vi "Main.vi"() -> ()   [LabVIEW 2015]
doc: "This template is for the Queued Message Handler design pattern.\n\nThe Event Handling Loop generates messages based on user interface actions.\n\nThe Message Handling Loop processes messages generated by the Event Handling Loop, or by other messages. The messages are string values, so new messages can be added easily to the Message Cases case structure in the Message Handling Loop. Each message cluster can also provide an optional value for Message Data, which is a variant that can be converted to whatever message-specific data is required."
uses:
  controls/UI Data.ctl
  support/Message Queue/Message Queue.lvlib
  support/User Event - Stop/User Event - Stop.lvlib
  support/Boiler System Globals.vi
  Boiler/Boiler.lvlib
  support/Notifiers/Notifiers.ctl
panel:
  out "Display <Replace Me>":string
  in  "Do Something Else <Replace Me>":bool
  in  "Do Something <Replace Me>":bool
  in  "Stop Button":bool
  # "These controls have associated \"Value Changed\" events configured in the Event Structure on the diagram.\n\nReplace them (and reconfigure the Event Structure) with the controls you need for your application."
  # "This template is for the Queued Message Handler design pattern.\n\nSee the block diagram for more information on how to use this template."
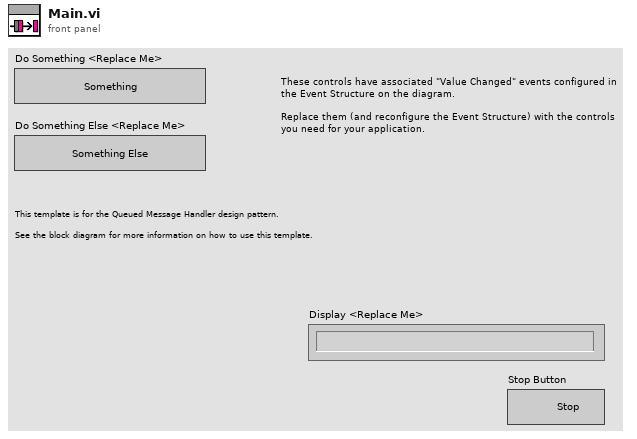
[diagram p1: front panel]
types:
  T1 = typedef "Notifiers.ctl" = cluster{"Handshake":refnum<notifier>, "Flame level":refnum<notifier>, "Controller exit":refnum<notifier>, "Boiler exit":refnum<notifier>}
  T2 = typedef "UI Data.ctl" = cluster{"Boolean <Replace Me>":bool, "String <Replace Me>":string, "Numeric <Replace Me>":dbl, "Do Something Ref":refnum<vi>, "Do Something Else Ref":refnum<vi>, "Data Display Ref":refnum<vi>, "Stop Button Ref":refnum<vi>}
  T3 = typedef "Message Queue.lvlib/All Message Queues.ctl" = cluster{"MHL":refnum<queue>, "Boiler Controller":refnum<queue>, "Boiler":refnum<queue>}
  T4 = enum32{"invalid app kind", "Development System", "Run Time System", "Student Edition", "Embedded LabVIEW", "Evaluation", "Custom"}
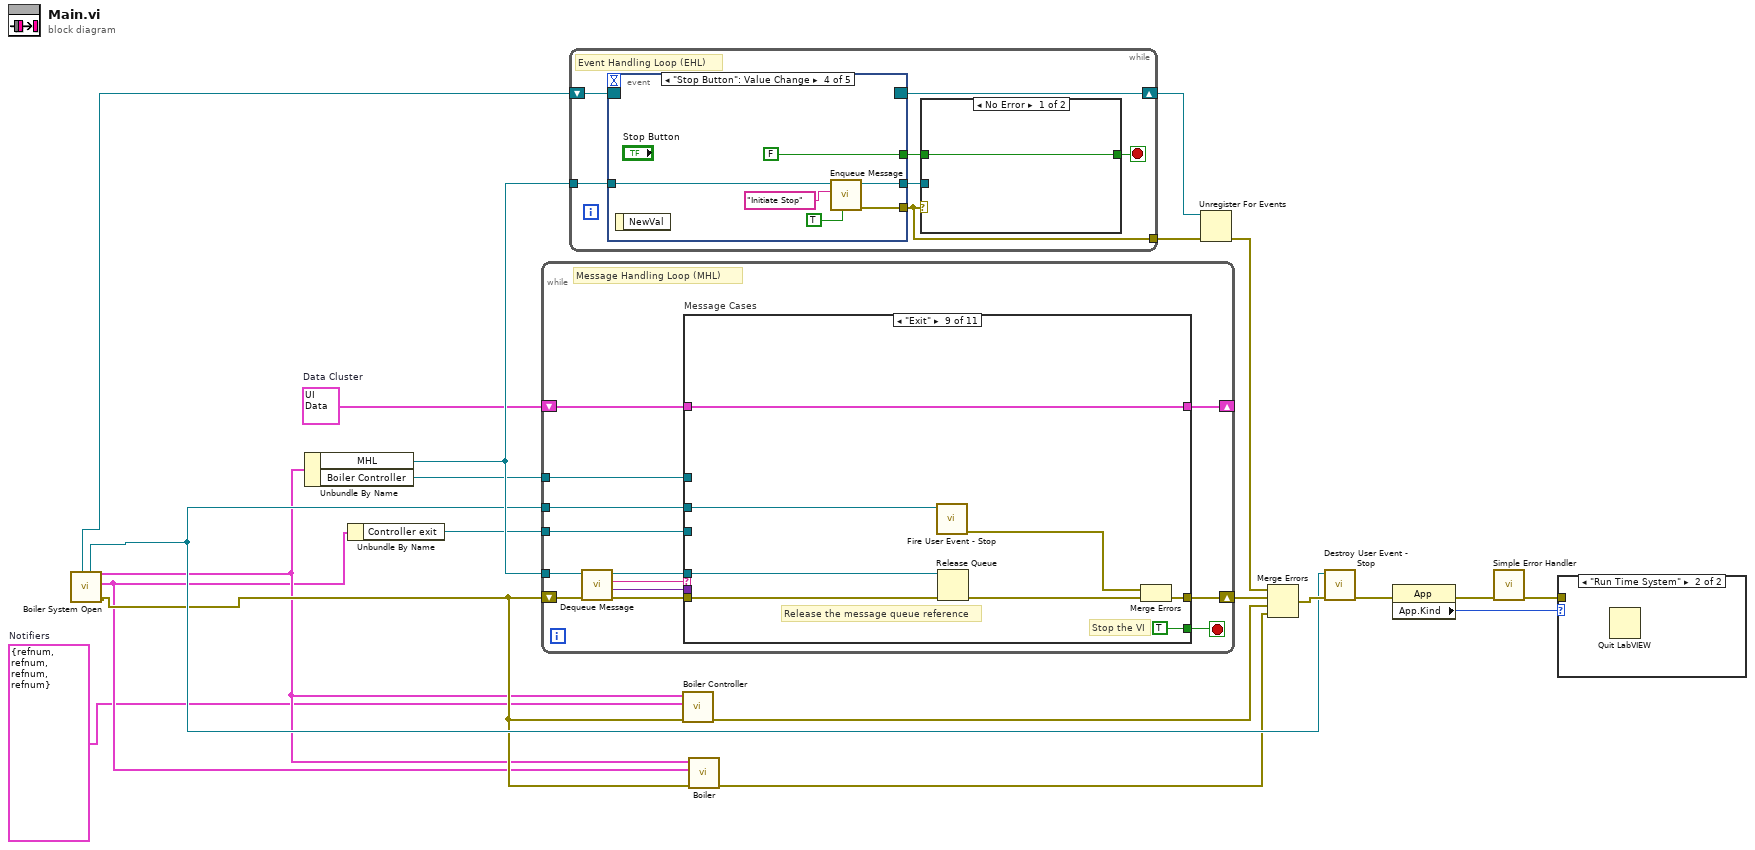
[diagram p0: block diagram]
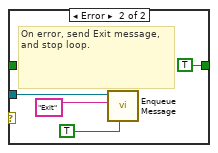
[diagram p3: hidden frame]
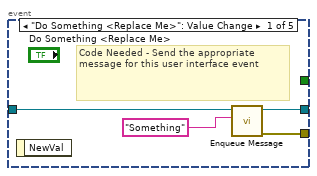
[diagram p4: hidden frame]
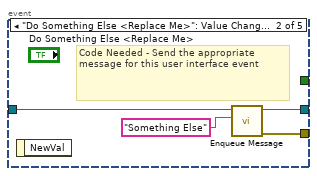
[diagram p5: hidden frame]
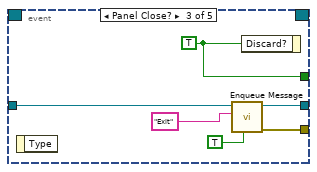
[diagram p6: hidden frame]
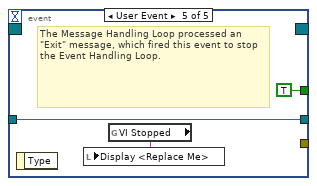
[diagram p7: hidden frame]
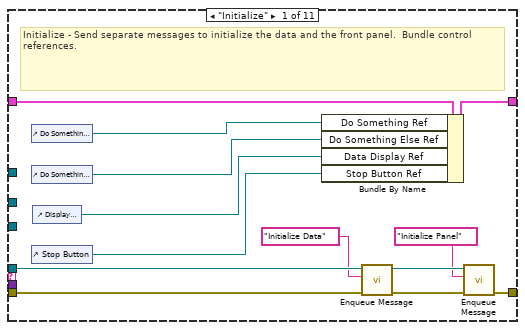
[diagram p8: hidden frame]
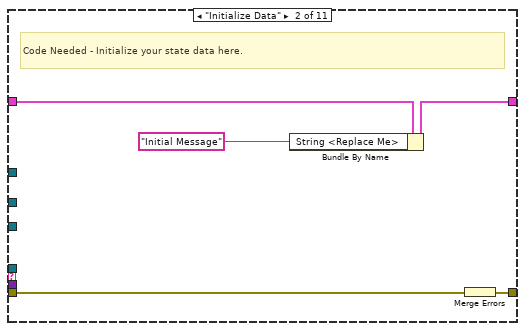
[diagram p9: hidden frame]
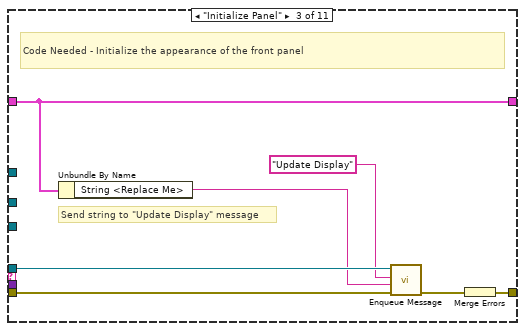
[diagram p10: hidden frame]
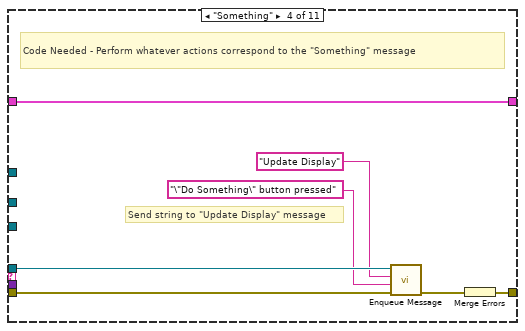
[diagram p11: hidden frame]
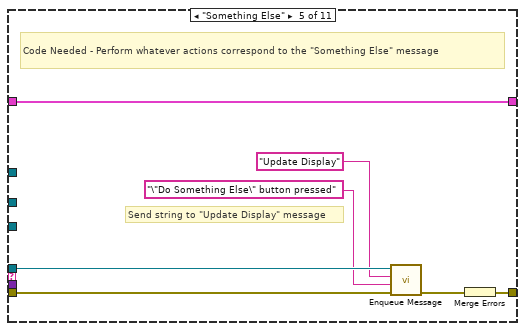
[diagram p12: hidden frame]
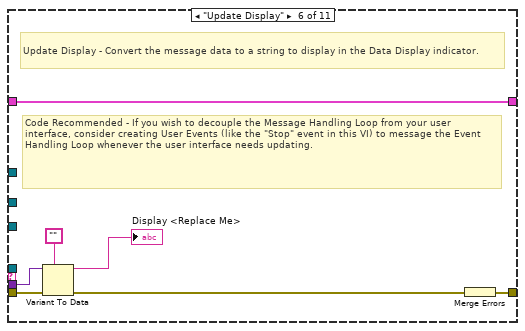
[diagram p13: hidden frame]
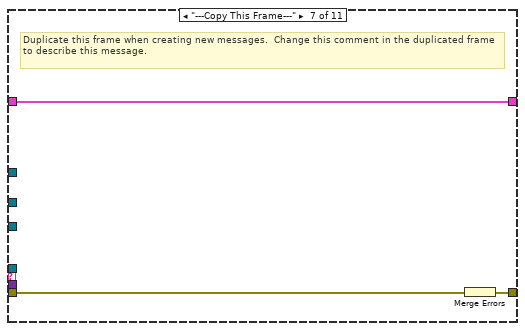
[diagram p14: hidden frame]
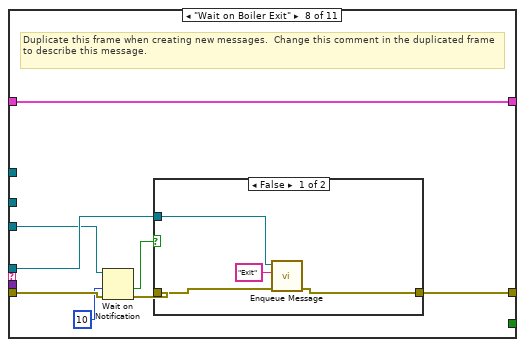
[diagram p15: hidden frame]
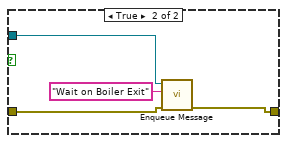
[diagram p16: hidden frame]
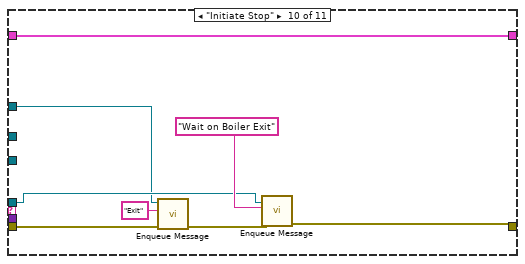
[diagram p17: hidden frame]
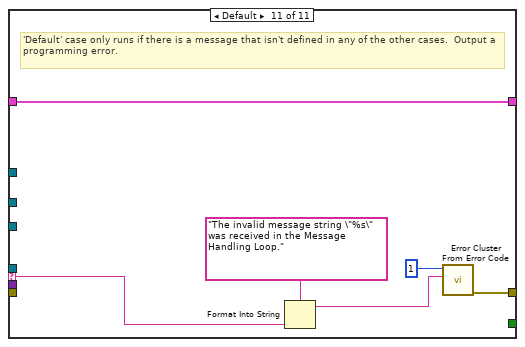
[diagram p18: hidden frame]
diagram:
  w1 = T1 {"Handshake"=refnum, "Flame level"=refnum, "Controller exit"=refnum, "Boiler exit"=refnum}  # Notifiers
  w14 = T2 {"Boolean <Replace Me>"=TRUE, "String <Replace Me>"="", "Numeric <Replace Me>"=0.0, "Do Something Ref"=refnum, "Do Something Else Ref"=refnum, "Data Display Ref"=refnum, "Stop Button Ref"=refnum}  # Data Cluster
  n1 = call "Boiler System Open.vi"() -> ("error out 2"=w6:errorcluster, "Notifiers"=w3:T1, "Message Queues out 2"=w5:T3, "User Event - Stop 2"=w7:refnum<user-event>, "Stop Event Registration Refnum 2"=w8:refnum<event-registration>)  [unwired: 7 in]
  n2 = Unbundle By Name(w5) -> ("MHL"=w20:refnum<queue>, "Boiler Controller"=w12:refnum<queue>)
  n3 = Unbundle By Name(w3) -> ("Controller exit"=w2:refnum<notifier>)
  n4 = while {
    tunnel: w20 -> [w24]
    shift-right: [w33] -> _
    shift-left: w14 -> [w34]
    tunnel: w7 -> [w30]
    shift-right: [w31] -> w21
    shift-left: w6 -> [w29]
    tunnel: w12 -> [w23]
    tunnel: w2 -> [w22]
    stop <- w32 stop-if-true
    # "Message Handling Loop (MHL)"
    n5 = call "Dequeue Message.vi"("error in (no error)"=w29, "Message Queue"=w24) -> ("error out"=w28:errorcluster, "Message Data"=w26:variant, "Message"=w27:string, "dup Message Queue"=w25:refnum<queue>)  [unwired: 6 in]
    n6 = case "Message Cases" shown="\"Exit\"" w27 {
      selector: w27 -> [_ _ _ _ _ _ _ _ _ _ w119]
      tunnel: w25 -> [w43 _ w56 w62 w69 _ _ w89 w107 w109 _]
      tunnel: w28 -> [w46 w52 w57 w64 w71 w78 w83 w88 w100 w114 _]
      tunnel: [w47 w48 w58 w65 w72 w79 w81 w90 w103 w112 w117] -> w31
      tunnel: w34 -> [w40 w51 w59 w66 w73 w80 w82 w91 w106 w115 w121]
      tunnel: [w39 w50 w59 w66 w73 w80 w82 w91 w106 w115 w121] -> w33
      tunnel: [_ _ _ _ _ _ _ _ TRUE _ _] -> w32
      tunnel: w26 -> [_ _ _ _ _ w77 _ _ _ _ _]
      tunnel: w30 -> [_ _ _ _ _ _ _ _ w102 _ _]
      tunnel: w23 -> [_ _ _ _ _ _ _ _ _ w108 _]
      tunnel: w22 -> [_ _ _ _ _ _ _ w85 _ _ _]
      frame "Initialize" {
        # "Initialize - Send separate messages to initialize the data and the front panel.  Bundle control references."
        n7 = control-ref of="Do Something <Replace Me>"() -> (w38:refnum<vi>)
        n8 = control-ref of="Do Something Else <Replace Me>"() -> (w37:refnum<vi>)
        n9 = control-ref of="Stop Button"() -> (w35:refnum<vi>)
        n10 = control-ref of="Display <Replace Me>"() -> (w36:refnum<vi>)
        n11 = Bundle By Name(cluster=w40, "Do Something Ref"=w38, "Do Something Else Ref"=w37, "Data Display Ref"=w36, "Stop Button Ref"=w35) -> (w39:T2)
        n12 = call "Enqueue Message.vi"("error in (no error)"=w46, "Message"="Initialize Data", "Message Queue"=w43) -> ("error out"=w45:errorcluster, "dup Message Queue"=w44:refnum<queue>)  [unwired: 7 in]
        n13 = call "Enqueue Message.vi"("error in (no error)"=w45, "Message"="Initialize Panel", "Message Queue"=w44) -> ("error out"=w47:errorcluster)  [unwired: 7 in, 1 out]
      }
      frame "Initialize Data" {
        # "Code Needed - Initialize your state data here."
        n14 = Bundle By Name(cluster=w51, "String <Replace Me>"="Initial Message" ("Initial Message")) -> (w50:T2)
        n15 = Merge Errors(w52) -> (w48:errorcluster)
      }
      frame "Initialize Panel" {
        # "Send string to \"Update Display\" message"
        # "Code Needed - Initialize the appearance of the front panel"
        n16 = Unbundle By Name(w59) -> ("String <Replace Me>"=w53:string)
        n17 = call "Enqueue Message.vi"("error in (no error)"=w57, "Message Data"=w53, "Message"="Update Display", "Message Queue"=w56) -> ("error out"=w55:errorcluster)  [unwired: 6 in, 1 out]
        n18 = Merge Errors(w55) -> (w58:errorcluster)
      }
      frame "Something" {
        # "Send string to \"Update Display\" message"
        # "Code Needed - Perform whatever actions correspond to the \"Something\" message"
        n19 = call "Enqueue Message.vi"("error in (no error)"=w64, "Message Data"="\"Do Something\" button pressed" ("\"Do Something\" button pressed"), "Message"="Update Display", "Message Queue"=w62) -> ("error out"=w63:errorcluster)  [unwired: 6 in, 1 out]
        n20 = Merge Errors(w63) -> (w65:errorcluster)
      }
      frame "Something Else" {
        # "Send string to \"Update Display\" message"
        # "Code Needed - Perform whatever actions correspond to the \"Something Else\" message"
        n21 = call "Enqueue Message.vi"("error in (no error)"=w71, "Message Data"="\"Do Something Else\" button pressed" ("\"Do Something Else\" button pressed"), "Message"="Update Display", "Message Queue"=w69) -> ("error out"=w70:errorcluster)  [unwired: 6 in, 1 out]
        n22 = Merge Errors(w70) -> (w72:errorcluster)
      }
      frame "Update Display" {
        # "Code Recommended - If you wish to decouple the Message Handling Loop from your user interface, consider creating User Events (like the \"Stop\" event in this VI) to message the Event Handling Loop whenever the user interface needs updating."
        # "Update Display - Convert the message data to a string to display in the Data Display indicator."
        n23 = Variant To Data(error in=w78, type="", Variant=w77) -> (data=→"Display <Replace Me>":string, error out=w75:errorcluster)
        n24 = Merge Errors(w75) -> (w79:errorcluster)
      }
      frame "---Copy This Frame---" {
        # "Duplicate this frame when creating new messages.  Change this comment in the duplicated frame to describe this message."
        n25 = Merge Errors(w83) -> (w81:errorcluster)
      }
      frame "Wait on Boiler Exit" {
        # "Duplicate this frame when creating new messages.  Change this comment in the duplicated frame to describe this message."
        n26 = Wait on Notification(notifier=w85, timeout in ms (-1)=10, error in (no error)=w88) -> (timed out?=w84:bool, error out=w87:errorcluster)  [unwired: 1 in, 2 out]
        n27 = case shown="False" w84 {
          tunnel: w87 -> [w95 w99]
          tunnel: [w94 w98] -> w90
          tunnel: w89 -> [w92 w96]
          frame False {
            n28 = call "Enqueue Message.vi"("error in (no error)"=w95, "Message"="Exit", "Message Queue"=w92) -> ("error out"=w94:errorcluster)  [unwired: 7 in, 1 out]
          }
          frame True {
            n29 = call "Enqueue Message.vi"("error in (no error)"=w99, "Message"="Wait on Boiler Exit", "Message Queue"=w96) -> ("error out"=w98:errorcluster)  [unwired: 7 in, 1 out]
          }
        }
      }
      frame "Exit" {
        # "Stop the VI"
        # "Release the message queue reference"
        n30 = call "Fire User Event - Stop.vi"("User Event - Stop"=w102) -> ("error out"=w101:errorcluster)  [unwired: 10 in]
        n31 = Release Queue(queue=w107, error in (no error)=w100) -> (error out=w104:errorcluster)  [unwired: 1 in, 2 out]
        n32 = Merge Errors(w101, w104) -> (w103:errorcluster)
      }
      frame "Initiate Stop" {
        n33 = call "Enqueue Message.vi"("error in (no error)"=w114, "Message"="Exit", "Message Queue"=w108) -> ("error out"=w113:errorcluster)  [unwired: 7 in, 1 out]
        n34 = call "Enqueue Message.vi"("error in (no error)"=w113, "Message"="Wait on Boiler Exit", "Message Queue"=w109) -> ("error out"=w112:errorcluster)  [unwired: 7 in, 1 out]
      }
      frame Default {
        # "'Default' case only runs if there is a message that isn't defined in any of the other cases.  Output a programming error."
        n35 = Format Into String(format string="The invalid message string \"%s\" was received in the Message Handling Loop." ("Unknown Message Error Text"), w119) -> (resulting string=w116:string)  [unwired: 2 in, 1 out]
        n36 = call <vilib>:"Error Cluster From Error Code.vi"("error message (\"\")"=w116, "error code (0)"=1) -> ("error out"=w117:errorcluster)  [unwired: 7 in]
      }
    }
  }
  n37 = while {
    tunnel: w20 -> [w128]
    tunnel: [w124] -> w16
    shift-right: [w122] -> w15
    shift-left: w8 -> [w123]
    stop <- w126 stop-if-true
    # "Event Handling Loop (EHL)"
    n38 = event shown="[3] \"Stop Button\": Value Change" {
      selector: w123 -> [_ _ _ _ _]
      dyn-events: [_ _ _ _ _] -> w122
      timeout: _ -> [_ _ _ _ _]
      tunnel: [_ _ w147 FALSE ("Discard?") TRUE ("Discard?")] -> w127
      tunnel: w128 -> [w137 w141 w146 w153 w156]
      tunnel: [w136 w139 w145 w152 _] -> w124
      tunnel: [w135 w140 w144 w150 w156] -> w125
      event "Do Something <Replace Me>": Value Change {
        # "Code Needed - Send the appropriate message for this user interface event"
        n39 = event-data() -> ()  [unwired: 1 in, 1 out]
        n40 = call "Enqueue Message.vi"("Message"="Something", "Message Queue"=w137) -> ("error out"=w136:errorcluster, "dup Message Queue"=w135:refnum<queue>)  [unwired: 8 in]
      }
      event "Do Something Else <Replace Me>": Value Change {
        # "Code Needed - Send the appropriate message for this user interface event"
        n41 = event-data() -> ()  [unwired: 1 in, 1 out]
        n42 = call "Enqueue Message.vi"("Message"="Something Else", "Message Queue"=w141) -> ("error out"=w139:errorcluster, "dup Message Queue"=w140:refnum<queue>)  [unwired: 8 in]
      }
      event Panel Close? {
        w147 = TRUE ("Discard?")
        n43 = event-data() -> ()  [unwired: 1 in, 1 out]
        n44 = call "Enqueue Message.vi"("Priority Message? (F)"=TRUE, "Message"="Exit", "Message Queue"=w146) -> ("error out"=w145:errorcluster, "dup Message Queue"=w144:refnum<queue>)  [unwired: 7 in]
        n45 = event-data("Discard?"=w147) -> ()  [unwired: 1 in, 1 out]
      }
      event "Stop Button": Value Change {
        n46 = event-data() -> ()  [unwired: 1 in, 1 out]
        n47 = call "Enqueue Message.vi"("Priority Message? (F)"=TRUE, "Message"="Initiate Stop", "Message Queue"=w153) -> ("error out"=w152:errorcluster, "dup Message Queue"=w150:refnum<queue>)  [unwired: 7 in]
      }
      event User Event {
        # "The Message Handling Loop processed an \"Exit\" message, which fired this event to stop the Event Handling Loop."
        n48 = event-data() -> ()  [unwired: 1 in, 1 out]
        n49 = global read "Boiler System Globals.vi" "VI Stopped"() -> (w154:string)
        n50 = local write "Display <Replace Me>"(w154) -> ()
      }
    }
    n51 = case shown="No Error" w124 {
      tunnel: [w129 TRUE ("Discard?")] -> w126
      tunnel: w127 -> [w129 _]
      tunnel: w125 -> [_ w132]
      frame No Error {
      }
      frame Error {
        # "On error, send Exit message, and stop loop."
        n52 = call "Enqueue Message.vi"("Priority Message? (F)"=TRUE, "Message"="Exit", "Message Queue"=w132) -> ()  [unwired: 7 in, 2 out]
      }
    }
  }
  n53 = call "Boiler Controller.vi"("error in"=w6, "Notifiers"=w1, "Message Queues"=w5) -> ("error out"=w13:errorcluster)  [unwired: 8 in]
  n54 = call "Boiler.vi"("error in"=w6, "Notifiers"=w3, "Message Queues"=w5) -> ("error out"=w4:errorcluster)  [unwired: 8 in]
  n55 = Unregister For Events(event registration refnum=w15, error in=w16) -> (error out=w17:errorcluster)
  n56 = Merge Errors(w17, w21, w13, w4) -> (w18:errorcluster)
  n57 = call "Destroy User Event - Stop.vi"("error in (no error)"=w18, "User Event - Stop"=w7) -> ("error out"=w19:errorcluster)  [unwired: 9 in]
  n58 = property class="App"(error in=w19) -> (error out=w11:errorcluster, "App.Kind"=w10:T4)  [unwired: 1 in, 1 out]
  n59 = call <vilib>:"Simple Error Handler.vi"("error in (no error)"=w11) -> ("error out"=w9:errorcluster)  [unwired: 4 in, 4 out]
  n60 = case shown="\"Run Time System\"" w10 {
    tunnel: w9 -> [_ _]
    frame Default {
    }
    frame "Run Time System" {
      n61 = Quit LabVIEW() -> ()  [unwired: 1 in]
    }
  }
